vi "pid tests.vi"() -> ()   [LabVIEW 2016]
panel:
  in  "dk 2":dbl=1.0 format="%#_13g"
  in  "pk 2":dbl=1.0 format="%#_13g"
  in  "ik 2":dbl=1.0 format="%#_13g"
  out "Waveform Graph 2":dbl[](graph)
  out "Waveform Graph":dbl[][](graph)
  in  "dk":dbl=1.0 format="%#_13g"
  in  "pk":dbl=1.0 format="%#_13g"
  in  "ik":dbl=1.0 format="%#_13g"
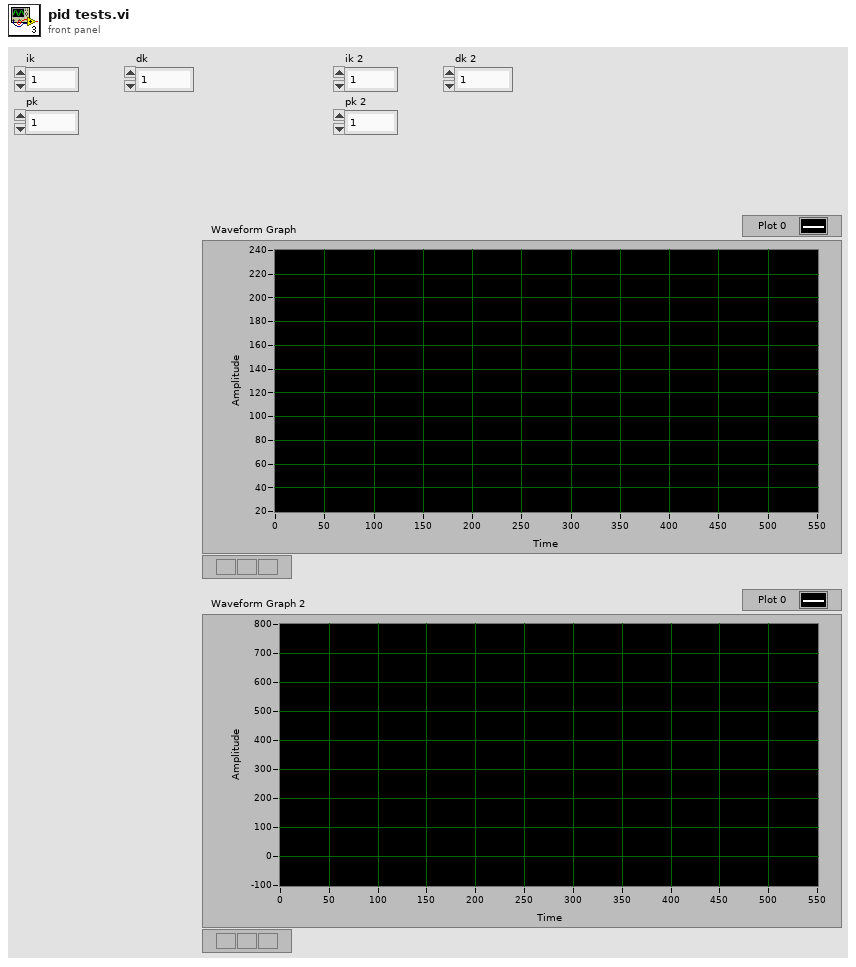
[diagram p1: front panel]
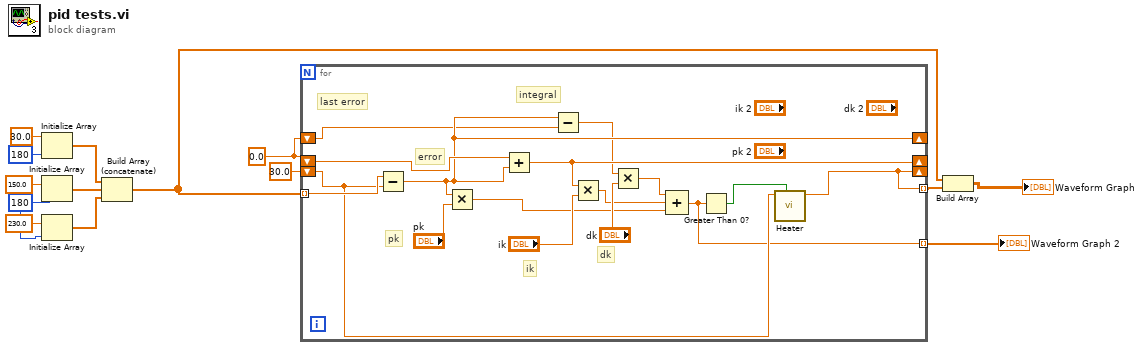
[diagram p0: block diagram]
diagram:
  w8 = 0.0
  w12 = 180 ("dimension size")
  n1 = Initialize Array(30.0 ("element"), 180 ("dimension size")) -> (w3:dbl[])
  n2 = Initialize Array(150.0 ("element"), w12) -> (w11:dbl[])
  n3 = Initialize Array(230.0 ("element"), w12) -> (w10:dbl[])
  n4 = Build Array (concatenate)(w3, w11, w10) -> (w5:dbl[])
  n5 = for {
    tunnel: w5 -> [w30] mode=indexing
    shift-right: [w16] -> _
    shift-left: 30.0 ("Temp out") -> [w17]
    shift-right: [w27] -> _
    shift-left: w8 -> [w28]
    shift-right: [w25] -> _
    shift-left: w8 -> [w24]
    tunnel: [w16] -> w7 mode=indexing
    tunnel: [w15] -> w1 mode=indexing
    # "dk"
    # "last error"
    # "ik"
    # "integral"
    # "pk"
    # "error"
    n6 = Subtract(x=w30, y=w17) -> (x-y=w25:dbl)
    n7 = Multiply(x=w25, y="pk") -> (x*y=w19:dbl)
    n8 = Add(x=w28, y=w25) -> (x+y=w27:dbl)
    n9 = Subtract(x=w25, y=w24) -> (x-y=w23:dbl)
    n10 = Multiply(x=w27, y="ik") -> (x*y=w20:dbl)
    n11 = Multiply(x=w23, y="dk") -> (x*y=w21:dbl)
    n12 = Compound Arithmetic op=ADD(w21, w20, w19) -> (w15:dbl)
    n13 = Greater Than 0?(x=w15) -> (x > 0?=w18:bool)
    n14 = call "Heater.vi"("ON"=w18, "Temp in"=w17) -> ("Temp out"=w16:dbl)  [unwired: 9 in]
  }
  "Waveform Graph 2" <- w1
  n15 = Build Array(w5, w7) -> (→"Waveform Graph":dbl[][])
